vi "UsrProfiles-Reinitialise.vi"(8 "error in":errorcluster) -> (0 "error out":errorcluster)   [LabVIEW 2017]
uses:
  Globals/gl_UsrProfiles globals.vi
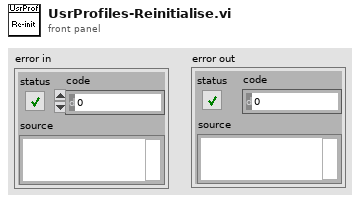
[diagram p1: front panel]
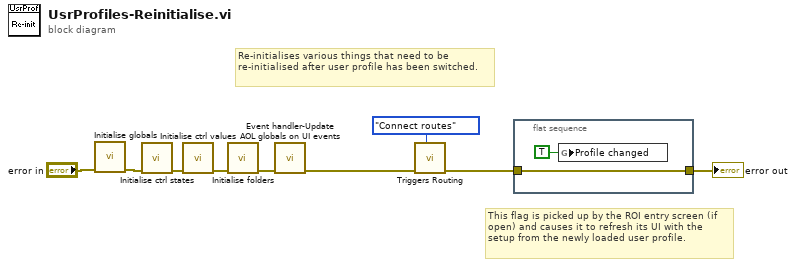
[diagram p0: block diagram]
diagram:
  # "This flag is picked up by the ROI entry screen (if open) and causes it to refresh its UI with the setup from the newly loaded user profile."
  # "Re-initialises various things that need to be re-initialised after user profile has been switched."
  n1 = call "Initialise globals.vi"("error in (no error)"="error in") -> ("error out"=w8:errorcluster)  [unwired: 10 in]
  n2 = call "Initialise ctrl states.vi"("error in (no error)"=w8) -> ("error out"=w7:errorcluster)  [unwired: 10 in]
  n3 = call "Initialise ctrl values.vi"("error in (no error)"=w7) -> ("error out"=w6:errorcluster)  [unwired: 10 in]
  n4 = call "Initialise folders.vi"("error in (no error)"=w6) -> ("error out"=w5:errorcluster)  [unwired: 10 in]
  n5 = call "Event handler-Update AOL globals on UI events.vi"("error in (no error)"=w5) -> ("error out"=w1:errorcluster)  [unwired: 10 in]
  n6 = call "Triggers Routing.vi"("Function"=enum16{"Connect routes", "Disconnect routes"}."Connect routes", "error in (no error)"=w1) -> ("error out (no error)"=w3:errorcluster)  [unwired: 9 in]
  n7 = flat-sequence {
    tunnel: w3 -> [w10]
    tunnel: [w10] -> w2
    frame #0 {
      n8 = global write "gl_UsrProfiles globals.vi" "Profile changed"(TRUE ("Profile changed")) -> ()
    }
  }
  "error out" <- w2
